vi "PFI-28000-Base_Get Overloads.vi"(8 "error in (no error)":errorcluster, 11 "PFI-28000-Base in":refnum<class "PFI-28000-Base.lvclass">) -> (0 "error out":errorcluster, 2 "Overloads":refnum<data-value>, 3 "PFI-28000-Base out":refnum<class "PFI-28000-Base.lvclass">)   [LabVIEW 2017, in "PFI-28000-Base.lvclass"]
uses:
  PFI-28000-Base.lvclass
  PFI-28000-Base.lvclass/PFI-28000-Base.ctl
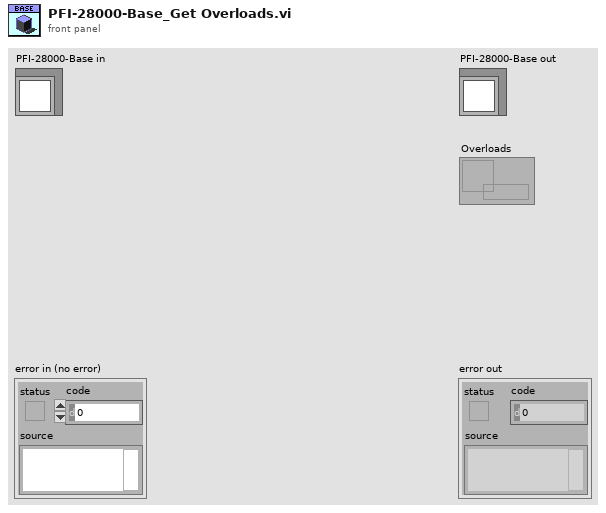
[diagram p1: front panel]
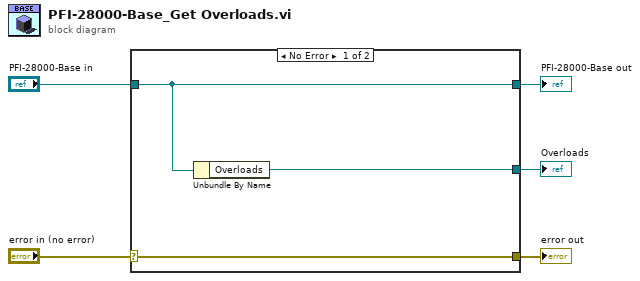
[diagram p0: block diagram]
diagram:
  n1 = case shown="No Error" "error in (no error)" {
    selector: "error in (no error)" -> [w8 w9]
    tunnel: [w8 w9] -> w4
    tunnel: [w7 w10] -> w2
    tunnel: "PFI-28000-Base in" -> [w7 w10]
    tunnel: [w6 _] -> w1
    frame No Error {
      n2 = Unbundle By Name(w7) -> ("Overloads"=w6:refnum<data-value>)
    }
    frame Error {
    }
  }
  "error out" <- w4
  "PFI-28000-Base out" <- w2
  "Overloads" <- w1
